vi "libssh2_session_handshake_tcp.vi"(8 "error in (no error)":errorcluster, 10 "tcp connection":refnum<k5>, 11 "session":T1) -> (0 "error out":errorcluster)   [LabVIEW 2017, in "libssh2.lvlib"]
doc: "Perform the SSH handshake on a session using a TCP connection.\n\nAfter handshake, verify the remote host key using libssh2_session_hostkey and libssh2_knownhost_checkp before any authentication."
uses:
  libssh2.lvlib
  Session Refnum.ctl
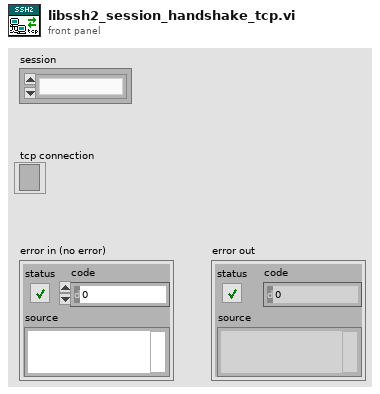
[diagram p1: front panel]
types:
  T1 = typedef "libssh2.lvlib/Session Refnum.ctl" = refnum<k1>
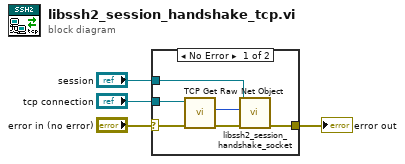
[diagram p0: block diagram]
diagram:
  n1 = case shown="No Error" "error in (no error)" {
    selector: "error in (no error)" -> [w7 w11]
    tunnel: [w5 w11] -> w4
    tunnel: "tcp connection" -> [w10 _]
    tunnel: "session" -> [w9 _]
    frame No Error {
      n2 = call <vilib>:"TCP Get Raw Net Object.vi"("error in (no error)"=w7, "connection ID"=w10) -> ("error out"=w6:errorcluster, "raw net object"=w8:u64)  [unwired: 7 in, 1 out]
      n3 = call "libssh2_session_handshake_socket.vi"("error in (no error)"=w6, "socket"=w8, "session"=w9) -> ("error out"=w5:errorcluster)  [unwired: 8 in]
    }
    frame Error {
    }
  }
  "error out" <- w4
